vi "AM Stopping Procedure.vi"(7 "Stop":bool, 8 "error in (no error)":errorcluster, 9 "Message Queues in":T1, 10 "Count":i32, 11 "Data Queue in":refnum<queue>) -> (0 "error out":errorcluster)   [LabVIEW 2020, in "Motion.lvlib"]
uses:
  Motion.lvlib
  support/Message Queue/All Message Queues.ctl
  support/Message Queue/Message Cluster.ctl
  support/Message Queue/Enqueue Message (Single).vi
  support/Message Queue/Message Queue.lvlib
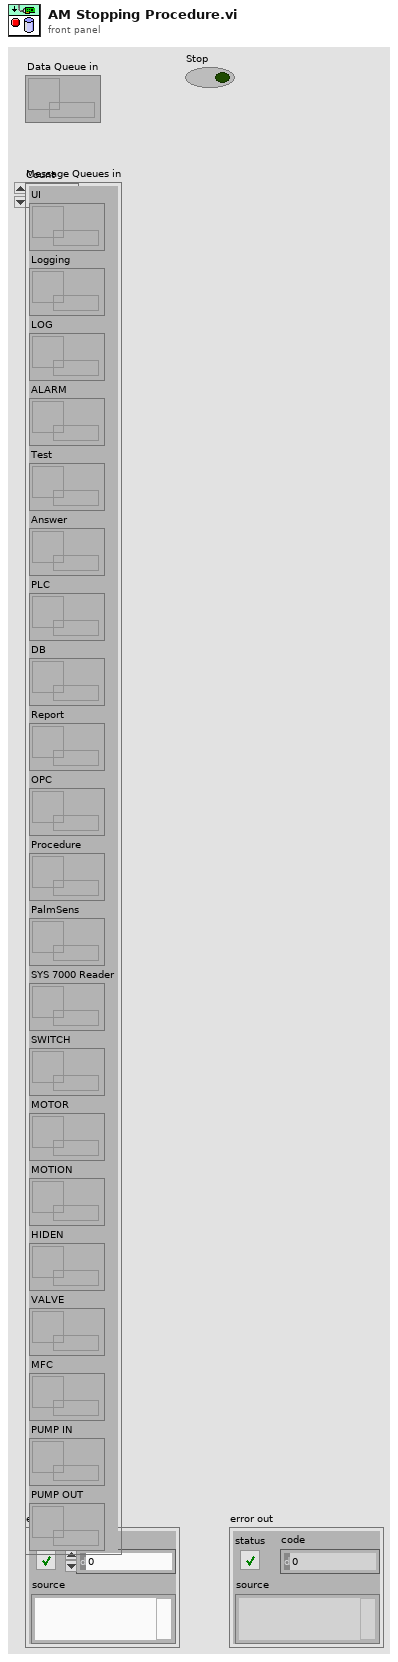
[diagram p1: front panel]
types:
  T1 = typedef "Message Queue.lvlib/All Message Queues.ctl" = cluster{"UI":refnum<queue>, "Logging":refnum<queue>, "LOG":refnum<queue>, "ALARM":refnum<queue>, "Test":refnum<queue>, "Answer":refnum<queue>, "PLC":refnum<queue>, "DB":refnum<queue>, "Report":refnum<queue>, "OPC":refnum<queue>, "Procedure":refnum<queue>, "PalmSens":refnum<queue>, "SYS 7000 Reader":refnum<queue>, "SWITCH":refnum<queue>, "MOTOR":refnum<queue>, "MOTION":refnum<queue>, "HIDEN":refnum<queue>, "VALVE":refnum<queue>, "MFC":refnum<queue>, "PUMP IN":refnum<queue>, "PUMP OUT":refnum<queue>}
  T2 = cluster{"Type CMD":string, "Mode CMD":string, "Main CMD":string}
  T3 = typedef "Message Queue.lvlib/Message Cluster.ctl" = cluster{"Message":string, "Message Data":variant}
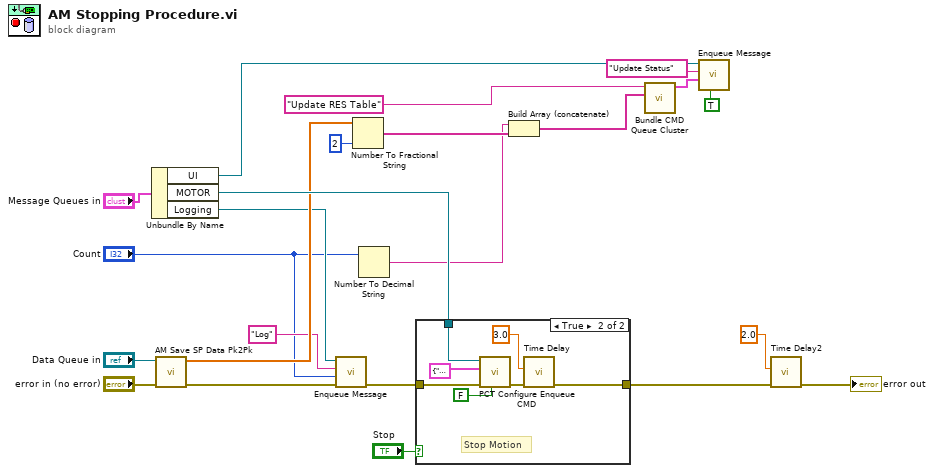
[diagram p0: block diagram]
diagram:
  n1 = Unbundle By Name("Message Queues in") -> ("UI"=w6:refnum<queue>, "MOTOR"=w23:refnum<queue>, "Logging"=w7:refnum<queue>)
  n2 = call "AM Save SP Data Pk2Pk.vi"("error in (no error)"="error in (no error)", "Data Queue in"="Data Queue in") -> ("error out"=w15:errorcluster, "Mean Data"=w17:dbl[])  [unwired: 8 in]
  n3 = call-poly "Enqueue Message.vi"("error in (no error)"=w15, "Message Data"="Count", "Message"="Log", "Message Queue"=w7) -> ("error out"=w9:errorcluster)  [unwired: 6 in, 1 out]
  n4 = Number To Fractional String(number=w17, precision (6)=i16 2) -> (F-format string=w19:string[])  [unwired: 2 in]
  n5 = Number To Decimal String(number="Count") -> (decimal integer string=w3:string)  [unwired: 1 in]
  n6 = case shown="True" "Stop" {
    tunnel: w23 -> [_ w31]
    tunnel: [w24 w30] -> w11
    tunnel: w9 -> [w24 w26]
    frame False {
    }
    frame True {
      # "Stop Motion"
      n7 = call "PCT Configure Enqueue CMD.vi"("Parameter Data"=FALSE, "error in (no error)"=w26, "CMD"=T2 {"Type CMD"="Start", "Mode CMD"="", "Main CMD"="Action-Status"}, "CMD Queue in"=w31) -> ("error out"=w28:errorcluster)  [unwired: 5 in, 2 out]
      n8 = call "Time Delay"("error in (no error)"=w28, "Delay Time (s)"=3.0) -> ("error out"=w30:errorcluster)  [unwired: 9 in]
    }
  }
  n9 = Build Array (concatenate)(w3, w19) -> (w4:string[])
  n10 = call "Bundle CMD Queue Cluster.vi"("Message Data"=w4, "Message"="Update RES Table" ("Type CMD")) -> ("Message Cluster"=w20:T3)  [unwired: 9 in]
  n11 = call-poly "Enqueue Message.vi"("Priority Message? (F)"=TRUE, "Message Data"=w20, "Message"="Update Status", "Message Queue"=w6) -> ()  [unwired: 6 in, 2 out]
  n12 = call "Time Delay2"("error in (no error)"=w11, "Delay Time (s)"=2.0) -> ("error out"=→"error out":errorcluster)  [unwired: 9 in]
